vi "Test Result Monitor.vi"() -> ()   [LabVIEW 2018]
uses:
  Classes/STDF File Parser/STDF File Parser.lvclass
  Classes/GRR Core/GRR Core.lvclass
  Classes/Result Display/Result Display.lvclass
panel:
  out "error out":errorcluster
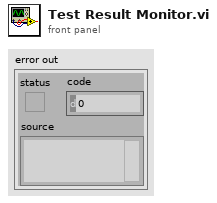
[diagram p1: front panel]
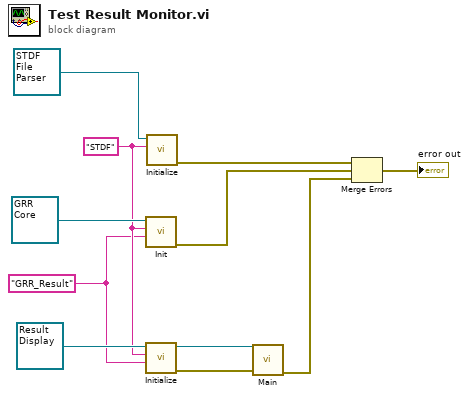
[diagram p0: block diagram]
diagram:
  w5 = "GRR_Result" ("GRR Result Session")
  w6 = "STDF" ("Parser Name")
  n1 = call "Init.vi"("GRR Result Session"=w5, "STDF Parser"=w6, "GRR Core in"=refnum<class "GRR Core.lvclass"> refnum ("GRR Core.lvclass")) -> ("error out"=w3:errorcluster)  [unwired: 7 in, 1 out]
  n2 = call "Initialize.vi"("GRR Data Mgr"=w5, "Test Data Mgr"=w6, "Result Display in"=refnum<class "Result Display.lvclass"> refnum) -> ("error out"=w8:errorcluster, "Result Display out"=w9:refnum<class "Result Display.lvclass">)  [unwired: 7 in]
  n3 = call "Initialize.vi"("Parser Name"=w6, "STDF File Parser in"=refnum<class "STDF File Parser.lvclass"> refnum ("STDF File Parser.lvclass")) -> ("error out"=w4:errorcluster)  [unwired: 8 in, 1 out]
  n4 = call "Main.vi"("error in (no error)"=w8, "Result Display in"=w9) -> ("error out"=w2:errorcluster)  [unwired: 8 in, 1 out]
  n5 = Merge Errors(w4, w3, w2) -> (→"error out":errorcluster)
